vi "Create Memory Buffer.vi"(8 "error in (no error)":errorcluster, 10 "size":u64 format="%d bytes", 11 "Buffer type":refnum<class "Memory Buffer.lvclass">) -> (0 "error out":errorcluster, 3 "Buffer out":refnum<class "Memory Buffer.lvclass">)   [LabVIEW 2017, in "Data Sharing Framework Engine.lvlib" / "Memory Buffer.lvclass"]
uses:
  Memory Buffer.lvclass
  C:/Program Files (x86)/National Instruments/LabVIEW 2017/vi.lib/National Instruments/Memory Manager/Classes/Pointer/Memory.Pointer.lvclass
  Memory Buffer.lvclass/Memory Buffer.ctl
  <vilib>/National Instruments/Memory Manager/Classes/Pointer/Memory.Pointer.lvclass/Memory.Pointer.ctl
  <vilib>/National Instruments/Memory Manager/Classes/Pointer/Memory.Pointer.New.1B.vi
  <vilib>/National Instruments/Memory Manager/Classes/Pointer/Memory.Pointer.Allocate.vi
  <vilib>/National Instruments/Memory Manager/Classes/Pointer/Memory.Pointer.Set Address.vi
  <vilib>/National Instruments/Memory Manager/Classes/Pointer/Memory.Pointer.Set Size.vi
  <vilib>/National Instruments/Memory Manager/Classes/Pointer/Memory.Pointer.Set Allocated.vi
  <vilib>/National Instruments/Memory Manager/Classes/Pointer/Memory.Pointer.lvclass
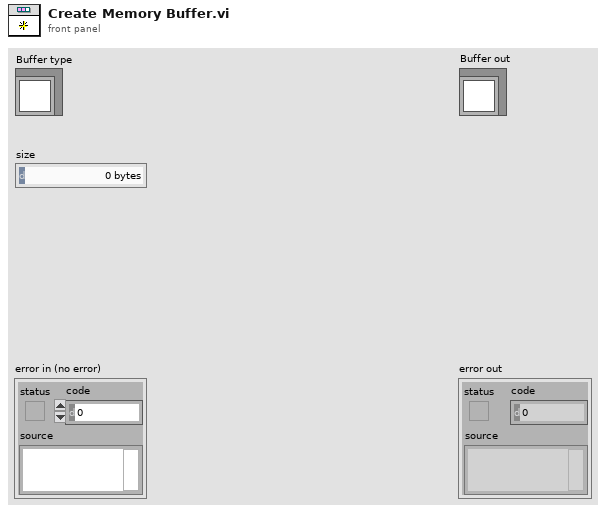
[diagram p1: front panel]
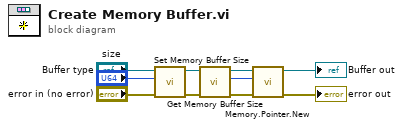
[diagram p0: block diagram]
diagram:
  n1 = call "Set Memory Buffer Size.vi"("buffer size"="size", "Buffer in"="Buffer type") -> ("Buffer out"=w3:refnum<class "Memory Buffer.lvclass">)  [unwired: 9 in]
  n2 = call "Get Memory Buffer Size.vi"("Buffer in"=w3) -> ("buffer size"=w1:u64, "Buffer out"=w2:refnum<class "Memory Buffer.lvclass">)  [unwired: 9 in]
  n3 = call-poly <vilib>:"Memory.Pointer.New.vi"("error in (no error)"="error in (no error)", "count (1)"=w1, "Pointer type"=w2) -> ("error out"=→"error out":errorcluster, "Pointer"=→"Buffer out":refnum<class "Memory Buffer.lvclass">)  [unwired: 7 in]
